vi "Queue Create.vi"(9 "Queue jettl":refnum<class "Queue jettl.lvclass">, 10 "Alias":string, 11 "Queue Create in":refnum<class "Queue Create.lvclass">) -> (3 "Queue Create out":refnum<class "Queue Create.lvclass">)   [LabVIEW 2021, in "jettl.lvlib" / "Queue Create.lvlib" / "Queue Create.lvclass"]
uses:
  Queue Create.lvclass
  jettl/Queue jettl/Queue jettl.lvclass
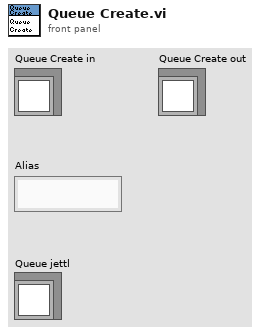
[diagram p1: front panel]
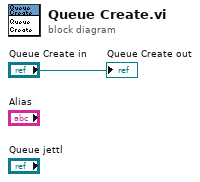
[diagram p0: block diagram]
diagram:
  "Queue Create out" <- "Queue Create in"
